vi "bell.vi"() -> ()   [LabVIEW 2014]
uses:
  <vilib>/MakerHub/LINX/Public/Peripherals/Digital/Digital Write 1 Chan.vi
  <vilib>/Analysis/1siggen.llb/Ramp Pattern by Samples.vi
  <vilib>/MakerHub/LINX/Public/Peripherals/Digital/Digital Write N Chans.vi
  <vilib>/MakerHub/LINX/Private/Local IO/LinxDigitalWrite.vi
  <vilib>/MakerHub/LINX/Public/Utilities/Check Channel.vi
  <vilib>/MakerHub/LINX/Private/Local IO/Handle Errors.vi
  <vilib>/MakerHub/LINX/Public/Utilities/Open Local.vi
  <vilib>/MakerHub/LINX/Private/Utilties/Generate Error.vi
  <vilib>/gmath/NI_Gmath.lvlib
  <vilib>/Analysis/NI_AALBase.lvlib
  <vilib>/MakerHub/LINX/LMH-LINX.lvlib
panel:
  in  "Digital Output Channel":u8=26
  in  "Stop Button":bool
  out "Loop Rate (Hz)":u32=4
  out "LED Value":bool=TRUE
  in  "Sound Format":T1={"sound quality"=enum."stereo", "rate"=44100} {"rate" min=4000 step=1000}
  out "Waveform Graph 2":dbl[](graph)
  out "Waveform Graph":dbl[](graph)
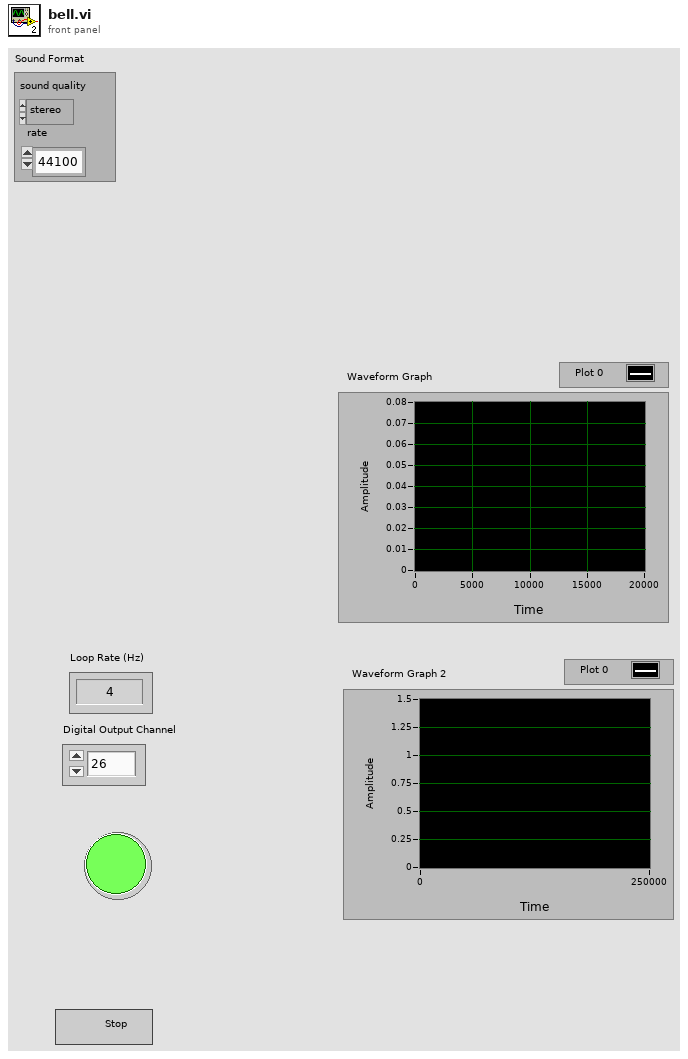
[diagram p1: front panel]
types:
  T1 = cluster{"sound quality":enum16{"mono", "stereo"}, "rate":u32}
  T2 = typedef "LMH-LINX.lvlib/LINX Ref.ctl" = cluster{"IO":T3, "Interface":T4, "LINX Device Config":T5}
  T3 = typedef "LMH-LINX.lvlib/Platform.ctl" = enum16{"Remote", "Local"}
  T4 = typedef "LMH-LINX.lvlib/Interface.ctl" = enum16{"Serial", "TCP"}
  T5 = typedef "LMH-LINX.lvlib/Device.lvlib/LINX Device Config.ctl" = cluster{"Interface":T4, "COM Port":refnum<visa-resource-name>, "TCP Configuration":T6, "Device Family":u8, "Device ID":u8, "Device Name":string, "TCP Ref":refnum<k5>, "Channels":T7}
  T6 = typedef "LMH-LINX.lvlib/Device.lvlib/TCP Config.ctl" = cluster{"IP Address":string, "Port":u16}
  T7 = typedef "LMH-LINX.lvlib/Channels.ctl" = cluster{"DI":u8[], "DO":u8[], "AI":u8[], "AO":u8[], "PWM":u8[], "QE":u8[], "UART":u8[], "I2C 2":u8[], "SPI":u8[], "CAN":u8[], "Servo":u8[], "AI Ref (V)":dbl, "AI Resolution (Bits)":u8, "AO Ref (V)":dbl, "AO Resolution (Bits)":u8}
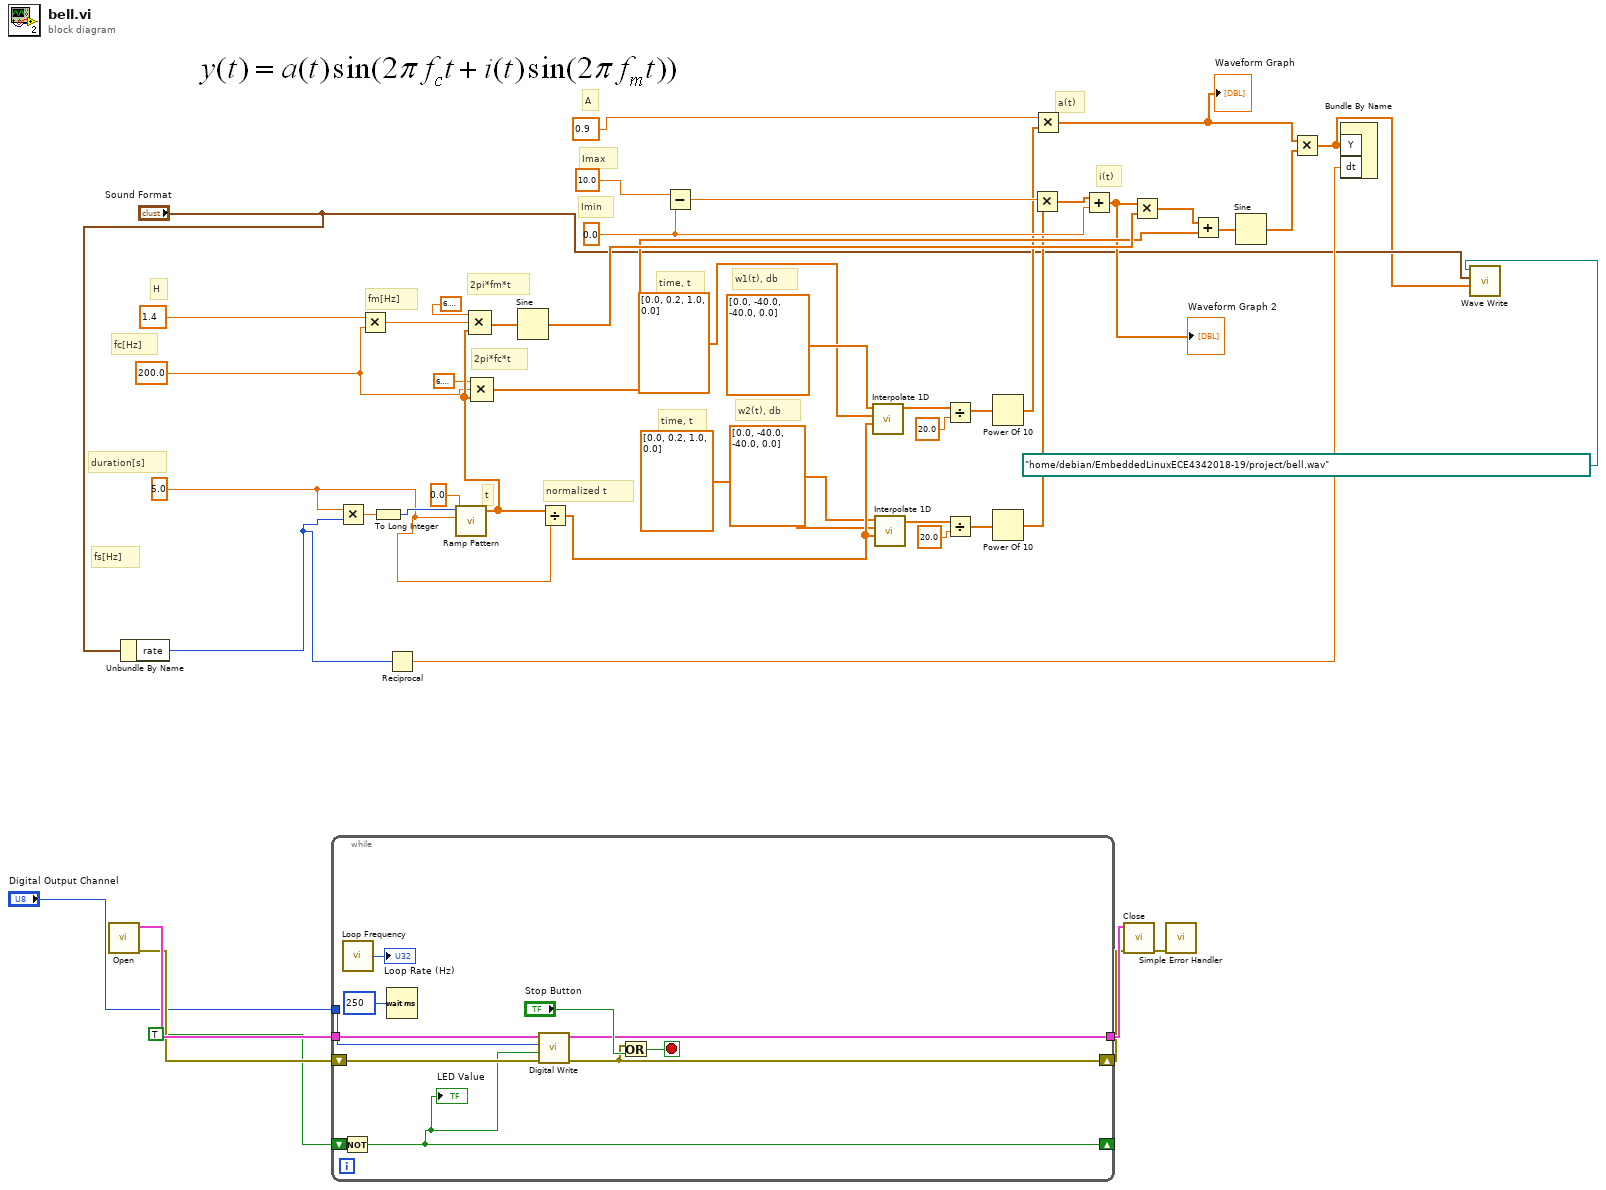
[diagram p0: block diagram]
diagram:
  w26 = 0.0 ("y")
  w41 = 5.0 ("x")
  w38 = 200.0 ("y")
  # "i(t)"
  # "a(t)"
  # "A"
  # "w1(t), db"
  # "time, t"
  # "w2(t), db"
  # "time, t"
  # "normalized t"
  # "Imin"
  # "Imax"
  # "2pi*fc*t"
  # "2pi*fm*t"
  # "t"
  # "fs[Hz]"
  # "duration[s]"
  # "fm[Hz]"
  # "fc[Hz]"
  # "H"
  n1 = call-poly <vilib>:"Open.vi"() -> ("Error Out"=w6:errorcluster, "LINX Resource"=w7:T2)  [unwired: 9 in, 1 out]
  n2 = Unbundle By Name("Sound Format") -> ("rate"=w9:u32)
  n3 = while {
    tunnel: w7 -> [w56]
    tunnel: [w55] -> w5
    shift-right: [w53] -> w4
    shift-left: w6 -> [w54]
    shift-right: [w49] -> _
    shift-left: TRUE -> [w50]
    tunnel: "Digital Output Channel" -> [w51]
    stop <- w59 stop-if-true
    n4 = Not(x=w50) -> (.not. x?=w49:bool)
    "LED Value" <- w49
    n5 = call <vilib>:"Loop Frequency.vi"() -> ("Loop Rate (Hz)"=→"Loop Rate (Hz)":u32)
    n6 = Wait (ms)(milliseconds to wait=u32 250) -> ()  [unwired: 1 out]
    n7 = call-poly <vilib>:"Digital Write.vi"("Error In"=w54, "Output Value"=w49, "DO Channel"=w51, "LINX Resource"=w56) -> ("Error Out"=w53:errorcluster, "LINX Resource"=w55:T2)  [unwired: 6 in]
    n8 = Or(x=w53, y="Stop Button") -> (x .or. y?=w59:bool)
  }
  n9 = Multiply(x=w41, y=w9) -> (x*y=w44:dbl)
  n10 = Multiply(x=1.4, y=w38) -> (x*y=w45:dbl)
  n11 = To Long Integer(number=w44) -> (32bit integer=w43:i32)
  n12 = Reciprocal(x=w9) -> (1/x=w20:dbl)
  n13 = call-poly <vilib>:"Ramp Pattern.vi"("start"=0.0, "end"=w41, "samples"=w43) -> ("Ramp Pattern"=w40:dbl[])  [unwired: 7 in, 1 out]
  n14 = Compound Arithmetic op=MULTIPLY(6.283185307179586, w45, w40) -> (w48:dbl[])
  n15 = Compound Arithmetic op=MULTIPLY(6.283185307179586, w38, w40) -> (w23:dbl[])
  n16 = Sine(x=w48) -> (sin(x)=w25:dbl[])
  n17 = Divide(x=w40, y=w41) -> (x/y=w36:dbl[])
  n18 = Subtract(x=10.0, y=w26) -> (x-y=w33:dbl)
  n19 = call <vilib>:"Interpolate 1D.vi"("xi"=w36, "X"=dbl[] [0.0, 0.2, 1.0, 0.0], "Y"=dbl[] [0.0, -40.0, -40.0, 0.0]) -> ("yi"=w35:dbl[])  [unwired: 6 in, 2 out]
  n20 = call <vilib>:"Interpolate 1D.vi"("xi"=w36, "X"=dbl[] [0.0, 0.2, 1.0, 0.0], "Y"=dbl[] [0.0, -40.0, -40.0, 0.0]) -> ("yi"=w34:dbl[])  [unwired: 6 in, 2 out]
  n21 = Divide(x=w35, y=20.0) -> (x/y=w14:dbl[])
  n22 = Divide(x=w34, y=20.0) -> (x/y=w15:dbl[])
  n23 = Power Of 10(x=w14) -> (10^x=w17:dbl[])
  n24 = Power Of 10(x=w15) -> (10^x=w16:dbl[])
  n25 = Multiply(x=w33, y=w16) -> (x*y=w27:dbl[])
  n26 = Multiply(x=0.9, y=w17) -> (x*y=w13:dbl[])
  "Waveform Graph" <- w13
  n27 = Add(x=w27, y=w26) -> (x+y=w12:dbl[])
  "Waveform Graph 2" <- w12
  n28 = call <vilib>:"Close.vi"("Error In"=w4, "LINX Resource"=w5) -> ("Error Out"=w3:errorcluster)  [unwired: 9 in]
  n29 = Multiply(x=w12, y=w25) -> (x*y=w24:dbl[])
  n30 = call <vilib>:"Simple Error Handler.vi"("error in (no error)"=w3) -> ()  [unwired: 4 in, 5 out]
  n31 = Add(x=w24, y=w23) -> (x+y=w22:dbl[])
  n32 = Sine(x=w22) -> (sin(x)=w21:dbl[])
  n33 = Multiply(x=w13, y=w21) -> (x*y=w8:dbl[])
  n34 = Bundle By Name("Y"=w8, "dt"=w20) -> ()  [unwired: 1 in, 1 out]
  n35 = call "Wave Write.vi"("Audio Input (+/- 1)"=w8, "Sound Format"="Sound Format", "File Path"=path "/home/debian/EmbeddedLinuxECE4342018-19/project/bell.wav" ("file path (use dialog)")) -> ()  [unwired: 8 in, 1 out]
